vi "ReadDB.vi"(8 "error in (no error)":errorcluster, 9 "index_item":i32, 10 "item_to_search":string, 11 "NameDB":string) -> (0 "error out":errorcluster, 2 "items_searched":string[][](array[string]))   [LabVIEW 2018]
doc: "Recopila toda la informacion de un .csv con separacion ( | ) y busca el item_to_search , en el indice de la columna seleccionada.\n\n - Retorna toda la informcion del elemento buscado"
uses:
  <vilib>/Utility/file.llb/Read Delimited Spreadsheet (string).vi
panel:
  out "index_item_to_search":i32[](array[numeric])
  out "all rows":string[][](array[string])
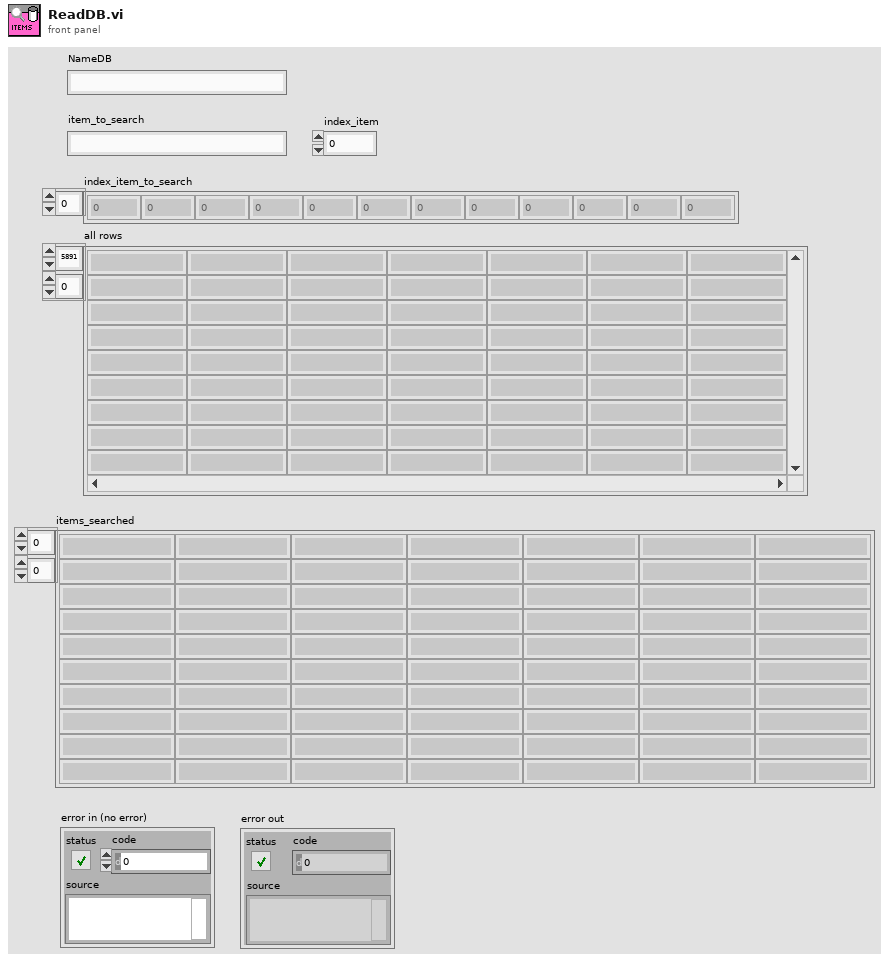
[diagram p1: front panel]
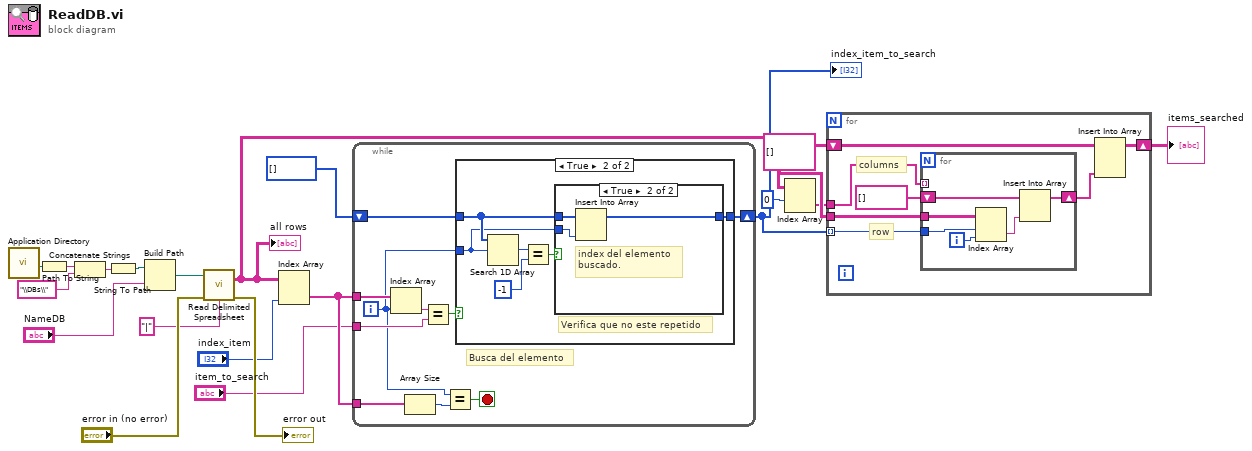
[diagram p0: block diagram]
diagram:
  n1 = call <vilib>:"Application Directory.vi"() -> ("Application Directory"=w20:path)
  n2 = Path To String(path=w20) -> (string=w19:string)
  n3 = Concatenate Strings(w19, "\\DBs\\") -> (w17:string)
  n4 = String To Path(string=w17) -> (path=w16:path)
  n5 = Build Path(base path=w16, name or relative path="NameDB") -> (appended path=w14:path)
  n6 = call-poly <vilib>:"Read Delimited Spreadsheet.vi"("file path (dialog if empty)"=w14, "error in (no error)"="error in (no error)", "delimiter (\\t)"="|" ("delimiter (\\t)")) -> ("all rows"=w7:string[][], "error out"=→"error out":errorcluster)  [unwired: 7 in, 4 out]
  "all rows" <- w7
  n7 = Index Array(array=w7, index (col)="index_item") -> (element=w9:string[])  [unwired: 1 in]
  n8 = while {
    shift-right: [w29] -> w10
    shift-left: i32[] [] -> [w30]
    tunnel: w9 -> [w28]
    tunnel: "item_to_search" -> [w26]
    tunnel: w9 -> [w24]
    i -> [w22]
    stop <- w21 stop-if-true
    # "Busca del elemento"
    n9 = Index Array(array=w28, index=w22) -> (element=w27:string)
    n10 = Array Size(array=w24) -> (size(s)=w23:i32)
    n11 = Equal?(x=w27, y=w26) -> (x = y?=w25:bool)
    n12 = Equal?(x=w22, y=w23) -> (x = y?=w21:bool)
    n13 = case shown="True" w25 {
      tunnel: w30 -> [w31 w35]
      tunnel: [w31 w33] -> w29
      tunnel: w22 -> [_ w32]
      frame False {
        # "No se encuentra"
      }
      frame True {
        # "Verifica que no este repetido"
        n14 = Search 1D Array(1D array=w35, element=w32) -> (index of element=w34:i32)  [unwired: 1 in]
        n15 = Equal?(x=w34, y=-1) -> (x = y?=w36:bool)
        n16 = case shown="True" w36 {
          tunnel: w35 -> [w38 w41]
          tunnel: [w38 w40] -> w33
          tunnel: w32 -> [_ w39]
          frame False {
          }
          frame True {
            # "index del elemento\nbuscado."
            n17 = Insert Into Array(array=w41, new element=w39) -> (w40:i32[])  [unwired: 1 in]
          }
        }
      }
    }
  }
  "index_item_to_search" <- w10
  n18 = Index Array(array=w7, index (row)=0) -> (element=w6:string[])  [unwired: 1 in]
  n19 = for {
    tunnel: w10 -> [w44] mode=indexing
    shift-right: [w47] -> w5
    shift-left: string[][] [] -> [w48]
    tunnel: w7 -> [w45]
    tunnel: w6 -> [w43]
    # "columns"
    # "row"
    n20 = for {
      shift-right: [w53] -> w42
      shift-left: string[] [] -> [w54]
      tunnel: w45 -> [w52]
      tunnel: w44 -> [w51]
      tunnel: w43 -> [_] mode=indexing
      i -> [w50]
      n21 = Index Array(array=w52, index (row)=w51, index (col)=w50) -> (element=w49:string)
      n22 = Insert Into Array(array=w54, new element=w49) -> (w53:string[])  [unwired: 1 in]
    }
    n23 = Insert Into Array(array=w48, new element=w42) -> (w47:string[][])  [unwired: 2 in]
  }
  "items_searched" <- w5
